vi "links.set.vi"(8 "error in":errorcluster, 10 "Links":T1, 11 "asset in":refnum<class "asset.lvclass">) -> (0 "error out":errorcluster, 3 "asset out":refnum<class "asset.lvclass">)   [LabVIEW 2020, in "asset.lvclass"]
uses:
  asset.lvclass
  nominal types/dataScope/links.ctl
  asset.lvclass/asset.ctl
  Nominal Client/Nominal Client.lvclass/Nominal Client.ctl
  Nominal Client/error.vi
  Nominal Client/trace.payload_sent.vi
  Nominal Client/trace.payload_received.vi
  Nominal Client/create.authorization_header.vi
  Nominal Client/error.vi/859f8e04-e495-489b-b5b4-7ac163f56130.vi
  Nominal Client/trace.calling_method.vi
  <vilib>/JDP Science/JDP Science Common Utilities/Trim Whitespace__JDP.vi
  <vilib>/AdvancedString/1D String Array to Delimited String.vi
  Nominal Client/api_token.get.vi
  <vilib>/JDP Science/JSONtext/support/Format JSON Object.vi
  <vilib>/Utility/libraryn.llb/Get File Extension.vi
  Nominal Client/log_file.write.vi
  <vilib>/JDP Science/JSONtext/Get all Object Items.vi
  <vilib>/Utility/error.llb/Error Cluster From Error Code.vi
  <vilib>/JDP Science/JSONtext/JSON text to Variant.vi
  <vilib>/JDP Science/JSONtext/LVClass Serializer/JSONtext LVClass Serializer.lvclass
  <vilib>/addons/_JKI.lib/REST Client/classes/Response Headers/Response Headers.lvclass
  <vilib>/addons/_JKI.lib/REST Client/classes/REST Client/REST Client.lvclass
  Nominal Client/Nominal Client.lvclass
  <vilib>/JDP Science/JSONtext/JSONtext.lvlib
  nominal types/dataScope/dataScopes.lvlib
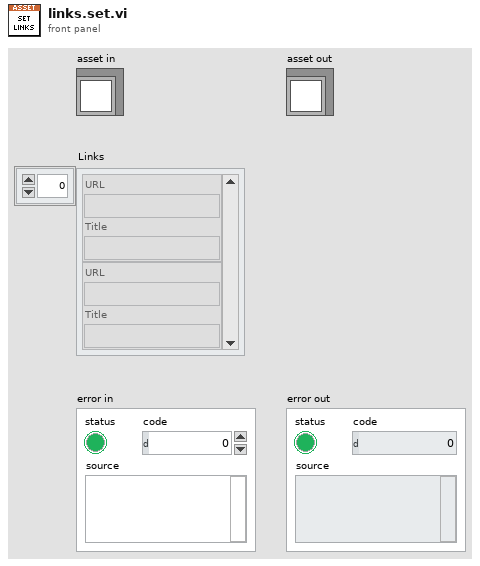
[diagram p1: front panel]
types:
  T1 = typedef "dataScopes.lvlib/links.ctl" = cluster{"URL":string, "Title":string}[]
  T2 = typedef "dataScopes.lvlib/data_scopes.ctl" = T3[]
  T3 = typedef "dataScopes.lvlib/data_scope.ctl" = cluster{"dataScopeName":string, "dataSource":T4, "seriesTags":map{string, string}, "offset":T6}
  T4 = typedef "dataScopes.lvlib/data_source.ctl" = cluster{"type":T5, "rid":string}
  T5 = typedef "dataScopes.lvlib/type.ctl" = enum16{"dataset", "connection", "logSet", "video"}
  T6 = typedef "dataScopes.lvlib/offset.ctl" = cluster{"seconds":i32, "nanos":i32, "picos":i32}
  T7 = cluster{"rid":string, "title":string, "properties":refnum<class "properties.lvclass">, "labels":refnum<class "labels.lvclass">, "Links":T1, "datascopes":T2, "createdAt":timestamp, "updatedAt":timestamp, "attachments":refnum<class "labels.lvclass">, "isStaged":bool, "isArchived":bool, "description":string, "createdBy":string, "type":string}
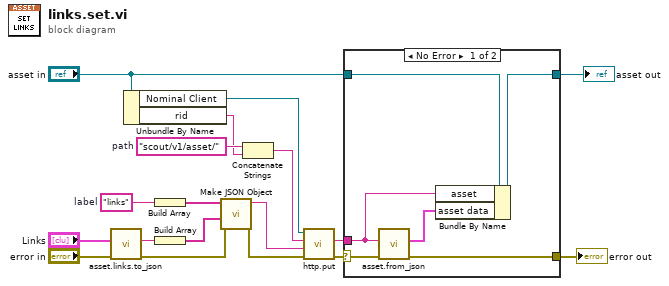
[diagram p0: block diagram]
diagram:
  w7 = "links"  # label
  w17 = "scout/v1/asset/"  # path
  n1 = call "asset.links.to_json.vi"("error in"="error in", "Links"="Links") -> ("error out"=w2:errorcluster, "json"=w1:string)  [unwired: 8 in]
  n2 = Unbundle By Name("asset in") -> ("Nominal Client"=w18:refnum<class "Nominal Client.lvclass">, "rid"=w15:string)
  n3 = Build Array(w7) -> (w8:string[])
  n4 = Build Array(w1) -> (w9:string[])
  n5 = call <vilib>:"Make JSON Object.vi"("error in (no error)"=w2, "JSON Items"=w9, "Item Names"=w8) -> ("error out"=w5:errorcluster, "<JSON>"=w6:string)  [unwired: 7 in]
  n6 = Concatenate Strings(w17, w15) -> (w16:string)
  n7 = call "http.put.vi"("error in"=w5, "Body"=w6, "Path"=w16, "Nominal Client in"=w18) -> ("error out"=w14:errorcluster, "Response"=w11:string)  [unwired: 4 in, 2 out]
  n8 = case shown="No Error" w14 {
    selector: w14 -> [w24 w26]
    tunnel: [w23 w26] -> w13
    tunnel: "asset in" -> [w22 w25]
    tunnel: w11 -> [w20 _]
    tunnel: [w19 w25] -> w10
    frame No Error {
      n9 = call "asset.from_json.vi"("error in"=w24, "asset"=w20) -> ("error out"=w23:errorcluster, "Asset Data"=w21:T7)  [unwired: 8 in]
      n10 = Bundle By Name(cluster=w22, "asset"=w20, "asset data"=w21) -> (w19:refnum<class "asset.lvclass">)
    }
    frame Error {
    }
  }
  "asset out" <- w10
  "error out" <- w13
